vi "Wariancja PBP.vi"(6 "Srednia N-1":dbl, 7 "wariancja N-1":dbl, 9 "Numeric":i32, 10 "Xn":dbl, 11 "Srednia":dbl) -> (3 "Wariancja":dbl)   [LabVIEW 2019]
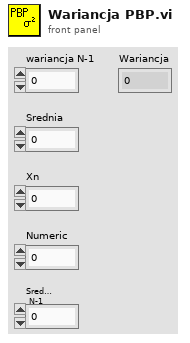
[diagram p1: front panel]
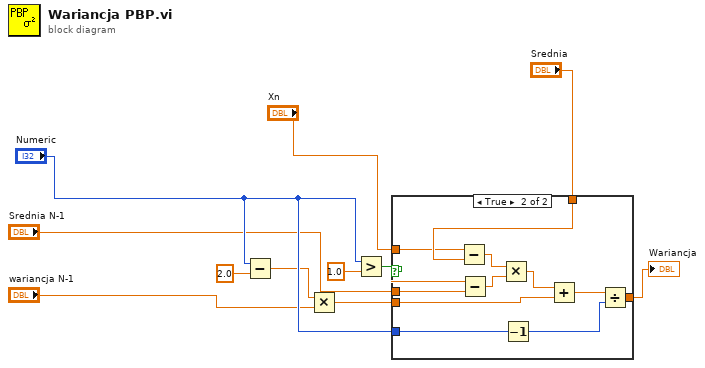
[diagram p0: block diagram]
diagram:
  n1 = Subtract(x="Numeric", y=2.0) -> (x-y=w10:dbl)
  n2 = Multiply(x=w10, y="wariancja N-1") -> (x*y=w6:dbl)
  n3 = Greater?(x="Numeric", y=1.0) -> (0:w8:bool)
  n4 = case shown="True" w8 {
    tunnel: "Srednia" -> [_ w23]
    tunnel: "Xn" -> [_ w22]
    tunnel: "Srednia N-1" -> [_ w21]
    tunnel: [w12 w16] -> w4
    tunnel: w6 -> [w12 w15]
    tunnel: "Numeric" -> [_ w13]
    frame False {
    }
    frame True {
      n5 = Subtract(x=w22, y=w23) -> (x-y=w20:dbl)
      n6 = Subtract(x=w22, y=w21) -> (x-y=w19:dbl)
      n7 = Multiply(x=w20, y=w19) -> (x*y=w18:dbl)
      n8 = Decrement(x=w13) -> (x-1=w14:i32)
      n9 = Add(x=w18, y=w15) -> (x+y=w17:dbl)
      n10 = Divide(x=w17, y=w14) -> (x/y=w16:dbl)
    }
  }
  "Wariancja" <- w4
